vi "SetCosts.vi"(11 "Start Goal Data":T1) -> (3 "Start Goal Data out":T1)   [LabVIEW 2013]
uses:
  Bug_StartGoalData.ctl
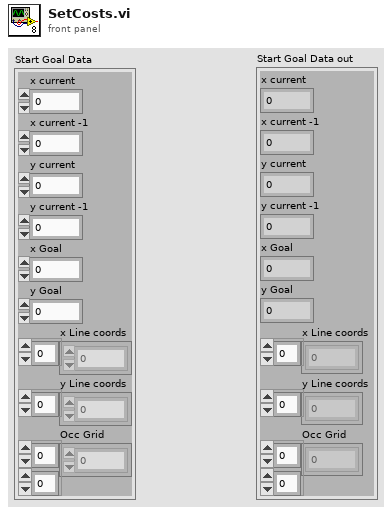
[diagram p1: front panel]
types:
  T1 = typedef "Bug_StartGoalData.ctl" = cluster{"x current":i32, "x current -1":i32, "y current":i32, "y current -1":i32, "x Goal":i32, "y Goal":i32, "x Line coords":i32[], "y Line coords":i32[], "Occ Grid":dbl[][]}
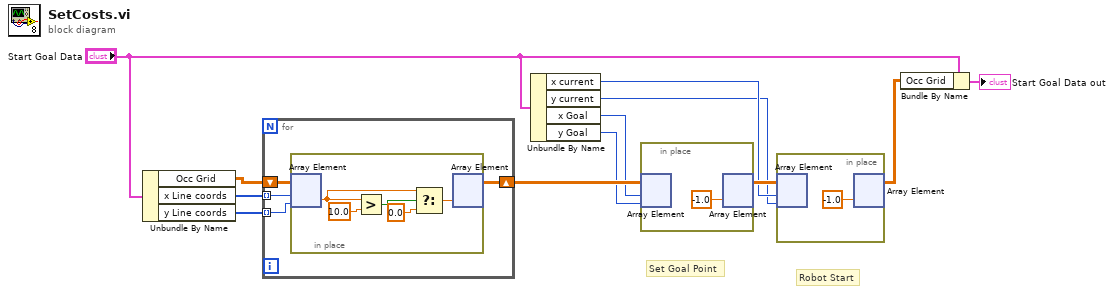
[diagram p0: block diagram]
diagram:
  # "Set Goal Point"
  # "Robot Start"
  n1 = Unbundle By Name("Start Goal Data") -> ("Occ Grid"=w6:dbl[][], "x Line coords"=w8:i32[], "y Line coords"=w7:i32[])
  n2 = for {
    tunnel: w8 -> [w15] mode=indexing
    tunnel: w7 -> [w14] mode=indexing
    shift-right: [w13] -> w12
    shift-left: w6 -> [w16]
    n3 = in-place {
      n4 = in-place-array #1(w16, w15, w14) -> (w18:dbl)
      n5 = Greater?(x=w18, y=10.0) -> (0:w20:bool)
      n6 = Select(t=w18, s=w20, f=0.0) -> (s? t:f=w19:dbl)
      n7 = in-place-array #1(w19) -> (w13:dbl[][])  [unwired: 2 out]
    }
  }
  n8 = Unbundle By Name("Start Goal Data") -> ("x current"=w10:i32, "y current"=w9:i32, "x Goal"=w4:i32, "y Goal"=w5:i32)
  n9 = in-place {
    n10 = in-place-array #2(w12, w4, w5) -> ()  [unwired: 1 out]
    n11 = in-place-array #2(-1.0) -> (w11:dbl[][])  [unwired: 2 out]
  }
  n12 = in-place {
    n13 = in-place-array #3(w11, w10, w9) -> ()  [unwired: 1 out]
    n14 = in-place-array #3(-1.0) -> (w1:dbl[][])  [unwired: 2 out]
  }
  n15 = Bundle By Name(cluster="Start Goal Data", "Occ Grid"=w1) -> (→"Start Goal Data out":T1)
